vi "ActionVIOnCompile.vi"(8 "error in (no error)":errorcluster, 11 "Device Item Ref in":T7 format="%.0x") -> (0 "error out":errorcluster)   [LabVIEW 2017, in "SLSC Switch System Explorer.lvlib"]
uses:
  SLSC Switch System Explorer.lvlib
  <vilib>/NI Veristand/Custom Device API/Custom Device Item Ref.ctl
  Shared/Compiled.Settings.ctl
  Shared/Communication Configuration.ctl
  Shared/Driver Configuration.ctl
  Shared/Endpoint Configuration Cluster.ctl
  Shared/Endpoint Configuration Enum.ctl
  Shared/FIFO Indices.ctl
  Shared/Constants.vi
  <vilib>/NI Veristand/Custom Device API/Set Item Property (Variant).vi
  <vilib>/NI Veristand/Custom Device API/Custom Device API.lvlib
  Shared/SLSC Switch Shared.lvlib
panel:
  out "output cluster":T1
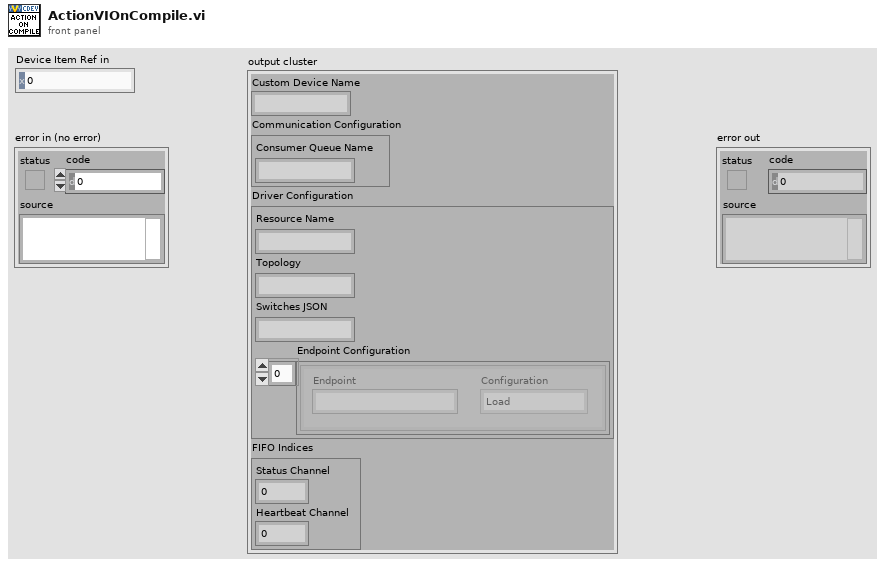
[diagram p1: front panel]
types:
  T1 = typedef "SLSC Switch Shared.lvlib/Compiled.Settings.ctl" = cluster{"Custom Device Name":string, "Communication Configuration":T2, "Driver Configuration":T3, "FIFO Indices":T6}
  T2 = typedef "SLSC Switch Shared.lvlib/Communication Configuration.ctl" = cluster{"Consumer Queue Name":string}
  T3 = typedef "SLSC Switch Shared.lvlib/Driver Configuration.ctl" = cluster{"Resource Name":string, "Topology":string, "Switches JSON":string, "Endpoint Configuration":T4[]}
  T4 = typedef "SLSC Switch Shared.lvlib/Endpoint Configuration Cluster.ctl" = cluster{"Endpoint":string, "Configuration":T5}
  T5 = typedef "SLSC Switch Shared.lvlib/Endpoint Configuration Enum.ctl" = enum16{"Load", "Source", "Configuration"}
  T6 = typedef "SLSC Switch Shared.lvlib/FIFO Indices.ctl" = cluster{"Status Channel":i32, "Heartbeat Channel":i32}
  T7 = typedef "Custom Device API.lvlib/Custom Device Item Ref.ctl" = u64
  T8 = typedef "Custom Device API.lvlib/Custom Device Item Info.ctl" = cluster{"Name":string, "Is Channel":bool, "GUID":string, "Is Waveform":bool}
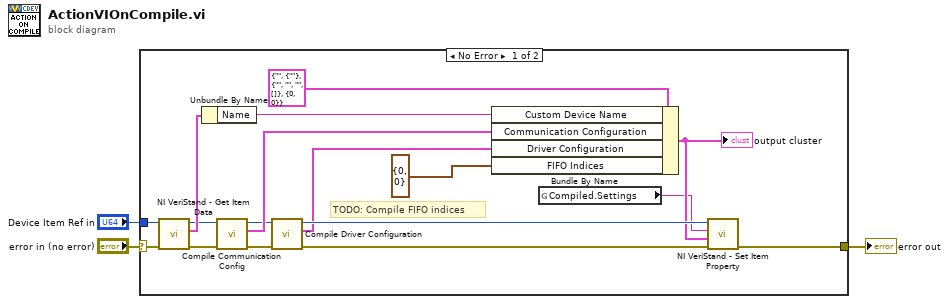
[diagram p0: block diagram]
diagram:
  n1 = case shown="No Error" "error in (no error)" {
    selector: "error in (no error)" -> [w19 w21]
    tunnel: [w20 w21] -> w2
    tunnel: "Device Item Ref in" -> [w18 _]
    frame No Error {
      # "TODO: Compile FIFO indices"
      n2 = call <vilib>:"NI VeriStand - Get Item Data.vi"("error in (no error)"=w19, "Item Ref in"=w18) -> ("error out"=w9:errorcluster, "Item Info"=w17:T8, "Item Ref out"=w10:T7)  [unwired: 6 in, 1 out]
      n3 = Unbundle By Name(w17) -> ("Name"=w16:string)
      n4 = call "Compile Communication Config.vi"("error in (no error)"=w9, "Device Ref in"=w10) -> ("error out"=w8:errorcluster, "Communication Configuration"=w7:T2, "Device Ref out"=w6:T7)  [unwired: 7 in]
      n5 = call "Compile Driver Configuration.vi"("error in (no error)"=w8, "Device Ref in"=w6) -> ("error out"=w14:errorcluster, "Driver Configuration"=w12:T3, "Device Ref out"=w13:T7)  [unwired: 7 in]
      n6 = Bundle By Name(cluster=T1 {"Custom Device Name"="", "Communication Configuration"={"Consumer Queue Name"=""}, "Driver Configuration"={"Resource Name"="", "Topology"="", "Switches JSON"="", "Endpoint Configuration"=[]}, "FIFO Indices"={"Status Channel"=0, "Heartbeat Channel"=0}} ("Compiled.Settings"), "Custom Device Name"=w16, "Communication Configuration"=w7, "Driver Configuration"=w12, "FIFO Indices"=T6 {"Status Channel"=0, "Heartbeat Channel"=0}) -> (w11:T1)
      "output cluster" <- w11
      n7 = global read "Constants.vi" "Compiled.Settings"() -> (w4:string)
      n8 = call-poly <vilib>:"NI VeriStand - Set Item Property.vi"("error in (no error)"=w14, "Value"=w11, "Property Name"=w4, "Item Ref in"=w13) -> ("error out"=w20:errorcluster)  [unwired: 5 in, 2 out]
    }
    frame Error {
    }
  }
  "error out" <- w2
